vi "Test Set Ignore Inherited Tests.vi"(8 "error in (no error)":errorcluster, 11 "Configuration Manager Test in":refnum<class "Configuration Manager Test.lvclass">) -> (0 "error out":errorcluster, 3 "Configuration Manager Test out":refnum<class "Configuration Manager Test.lvclass">)   [LabVIEW 2020, in "Configuration Manager Test.lvclass"]
uses:
  Configuration Manager Test.lvclass
  Configuration Manager Test.lvclass/Configuration Manager Test.ctl
  source/User Interface/Configuration Manager/Configuration Manager.lvclass
  <vilib>/Astemes/LUnit/Test Case.lvclass
  C:/Program Files (x86)/National Instruments/LabVIEW 2020/vi.lib/Astemes/LUnit/Test Case.lvclass
  C:/git/astemes-lunit/tests/Configuration Manager Test/Configuration Manager Test.lvclass
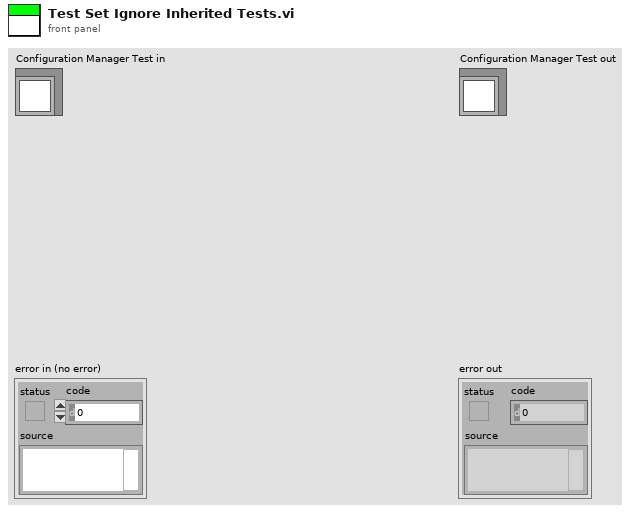
[diagram p1: front panel]
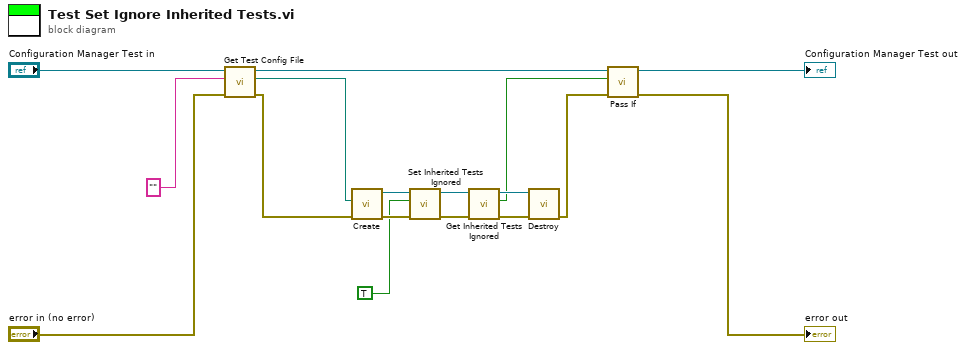
[diagram p0: block diagram]
diagram:
  n1 = call "Get Test Config File.vi"("error in (no error)"="error in (no error)", "File Content"="", "Configuration Manager Test in"="Configuration Manager Test in") -> ("error out"=w11:errorcluster, "File Path"=w5:path, "Configuration Manager Test out"=w8:refnum<class "Configuration Manager Test.lvclass">)  [unwired: 6 in]
  n2 = call "Create.vi"("error in (no error)"=w11, "configuration file path"=w5) -> ("error out"=w14:errorcluster, "Configuration Manager out"=w3:refnum<class "Configuration Manager.lvclass">)  [unwired: 8 in]
  n3 = call "Set Inherited Tests Ignored.vi"("error in (no error)"=w14, "Ingore Inherited?"=TRUE, "Configuration Manager In"=w3) -> ("error out"=w4:errorcluster, "Configuration Manager Out"=w2:refnum<class "Configuration Manager.lvclass">)  [unwired: 7 in]
  n4 = call "Get Inherited Tests Ignored.vi"("error in (no error)"=w4, "Configuration Manager In"=w2) -> ("error out"=w12:errorcluster, "Ignore Inherited?"=w6:bool, "Configuration Manager Out"=w13:refnum<class "Configuration Manager.lvclass">)  [unwired: 7 in]
  n5 = call "Destroy.vi"("error in (no error)"=w12, "Configuration Manager In"=w13) -> ("error out"=w10:errorcluster)  [unwired: 9 in]
  n6 = call <vilib>:"Pass If.vi"("error in (no error)"=w10, "Pass?"=w6, "LUnit Test Case In"=w8) -> ("error out"=→"error out":errorcluster, "LUnit Test Case Out"=→"Configuration Manager Test out":refnum<class "Configuration Manager Test.lvclass">)  [unwired: 7 in]
